vi "VL6180 Example.vi"() -> ()   [LabVIEW 2014]
uses:
  <vilib>/myRIO/Instrument Drivers/Onboard IO/DIO/typedefs/DIO Reference.ctl
  <vilib>/myRIO/Common/Instrument Driver Framework/Utilities/typedefs/myRIO Generic Hardware Reference.ctl
  <vilib>/myRIO/Common/Instrument Driver Framework/Utilities/typedefs/Hardware Version Enum.ctl
  <vilib>/myRIO/Common/Instrument Driver Framework/Utilities/typedefs/myRIO v1.0 Reference.ctl
  <vilib>/myRIO/Common/Instrument Driver Framework/Utilities/typedefs/Generic FPGA Reference.ctl
  <vilib>/myRIO/Common/Instrument Driver Framework/myRIO v1.0/DIO/typedefs/DIO Channels List.ctl
  <vilib>/myRIO/Common/Instrument Driver Framework/myRIO v1.0/DIO/typedefs/DIO Channels Enum.ctl
  <vilib>/userdefined/High Color/nirio_resource_hc.ctl
  <vilib>/myRIO/Common/Instrument Driver Framework/Utilities/vis/Is FPGA Ref Available.vi
  <vilib>/myRIO/Common/Instrument Driver Framework/myRIO v1.0/DIO/vis/myRIO v1.1 Open DIO.vi
  <vilib>/myRIO/Instrument Drivers/Onboard IO/DIO/vis/Write.vi
  <vilib>/myRIO/Common/Instrument Driver Framework/Utilities/vis/Validate Channels.vi
  <vilib>/myRIO/Common/Instrument Driver Framework/myRIO v1.0/DIO/vis/myRIO v1.0 Reserve DIO.vi
  <vilib>/myRIO/Common/Instrument Driver Framework/myRIO v1.0/Resource Manager/vis/myRIO v1.0 Reserve Channel List.vi
  <vilib>/myRIO/Common/Instrument Driver Framework/myRIO v1.0/DIO/vis/myRIO v1.0 Build MUX Configuration DIO.vi
  <vilib>/myRIO/Common/Instrument Driver Framework/myRIO v1.0/Resource Manager/vis/myRIO v1.0 Reserve Channel.vi
  <vilib>/myRIO/Common/Instrument Driver Framework/myRIO v1.0/Resource Manager/vis/myRIO v1.0 Unreserve Channel.vi
  <vilib>/myRIO/Common/Instrument Driver Framework/myRIO v1.0/Resource Manager/vis/myRIO v1.0 Create Configuration List.vi
  <vilib>/myRIO/Common/Instrument Driver Framework/myRIO v1.0/Resource Manager/vis/myRIO v1.0 Build Mutex Name.vi
  <vilib>/Utility/VariantDataType/GetNumericInfo.vi
  <vilib>/Utility/error.llb/Error Cluster From Error Code.vi
  <vilib>/myRIO/Common/Instrument Driver Framework/myRIO v1.0/myRIO v1.1 Open.vi
  <vilib>/myRIO/Common/Instrument Driver Framework/Utilities/vis/IO Manager.vi
  <vilib>/myRIO/Common/Instrument Driver Framework/Utilities/vis/Configuration Manager.vi
  <vilib>/myRIO/Common/Instrument Driver Framework/myRIO v1.0/Resource Manager/vis/myRIO v1.0 Configure IO.vi
  <vilib>/myRIO/Common/Instrument Driver Framework/myRIO v1.0/myRIO v1.0 Close.vi
  <vilib>/myRIO/Common/Instrument Driver Framework/myRIO v1.0/DIO/vis/myRIO v1.0 Write DIO.vi
  <vilib>/MakerHub/LINX/Public/Utilities/Open Local.vi
  <vilib>/myRIO/Express VI/Onboard IO/DO/DO Express VI.xnode
  <vilib>/myRIO/Instrument Drivers/Onboard IO/DIO/vis/myRIO DIO Open.xnode
  <vilib>/myRIO/Instrument Drivers/Onboard IO/DIO/DIO.lvlib
  <vilib>/MakerHub/LINX/LMH-LINX.lvlib
panel:
  in  "milliseconds to wait":u32
  in  "ToF 1 PWR":bool
  out "error out":errorcluster {"code" format="%.0x"}
  out "Sensor Error Code":u8
  out "Distance (mm)":u8
  in  "stop":bool
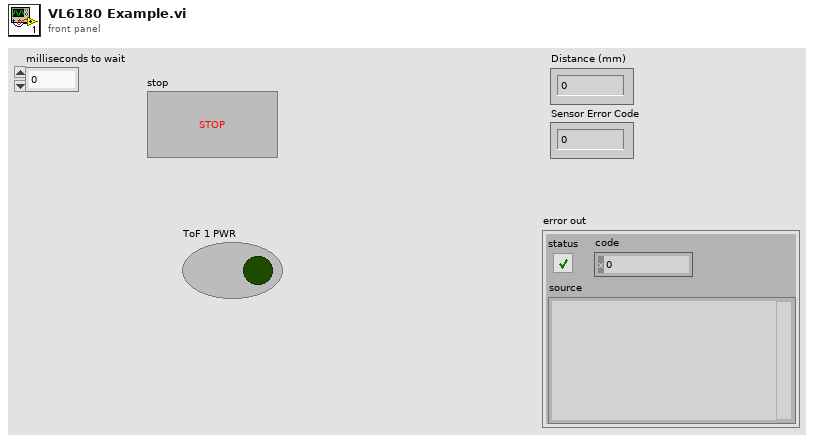
[diagram p1: front panel]
types:
  T1 = typedef "LMH-LINX.lvlib/LINX Ref.ctl" = cluster{"IO":T2, "Interface":T3, "LINX Device Config":T4}
  T2 = typedef "LMH-LINX.lvlib/Platform.ctl" = enum16{"Remote", "Local"}
  T3 = typedef "LMH-LINX.lvlib/Interface.ctl" = enum16{"Serial", "TCP"}
  T4 = typedef "LMH-LINX.lvlib/Device.lvlib/LINX Device Config.ctl" = cluster{"Interface":T3, "COM Port":refnum<visa-resource-name>, "TCP Configuration":T5, "Device Family":u8, "Device ID":u8, "Device Name":string, "TCP Ref":refnum<k5>, "Channels":T6}
  T5 = typedef "LMH-LINX.lvlib/Device.lvlib/TCP Config.ctl" = cluster{"IP Address":string, "Port":u16}
  T6 = typedef "LMH-LINX.lvlib/Channels.ctl" = cluster{"DI":u8[], "DO":u8[], "AI":u8[], "AO":u8[], "PWM":u8[], "QE":u8[], "UART":u8[], "I2C 2":u8[], "SPI":u8[], "CAN":u8[], "Servo":u8[], "AI Ref (V)":dbl, "AI Resolution (Bits)":u8, "AO Ref (V)":dbl, "AO Resolution (Bits)":u8}
  T7 = typedef "VL6180 Resource.ctl" = cluster{"I2C Channel":u8, "I2C Slave Address":u8, "Online":bool}
  T8 = typedef "DIO.lvlib/DIO Reference.ctl" = cluster{"myRIO Reference":T9, "DIO Channels List":T13}
  T9 = typedef "myRIO Generic Hardware Reference.ctl" = cluster{"myRIO Model":T10, "myRIO Hardware Reference":T11}
  T10 = typedef "Hardware Version Enum.ctl" = enum16{"Unknown", "myRIO-1900", "myRIO-1950"}
  T11 = typedef "myRIO v1.0 Reference.ctl" = cluster{"Generic FPGA Reference":T12, "Allow multiple opens":bool}
  T12 = typedef "Generic FPGA Reference.ctl" = refnum<k20>
  T13 = typedef "DIO Channels List.ctl" = T14[]
  T14 = typedef "DIO Channels Enum.ctl" = enum16{"Not Connected", "C/DIO0", "C/DIO1", "C/DIO2", "C/DIO3", "C/DIO4", "C/DIO5", "C/DIO6", "C/DIO7", "A/DIO0", "A/DIO1", "A/DIO2", "A/DIO3", "A/DIO4", "A/DIO5", "A/DIO6", "A/DIO7", "A/DIO8", "A/DIO9", "A/DIO10", "A/DIO11", "A/DIO12", "A/DIO13", "A/DIO14", "A/DIO15", "B/DIO0", "B/DIO1", "B/DIO2", "B/DIO3", "B/DIO4", "B/DIO5", "B/DIO6", "B/DIO7", "B/DIO8", "B/DIO9", "B/DIO10", "B/DIO11", "B/DIO12", "B/DIO13", "B/DIO14", "B/DIO15", "LED0", "LED1", "LED2", "LED3", "Button0"}
  T15 = typedef "nirio_resource_hc.ctl" = tag
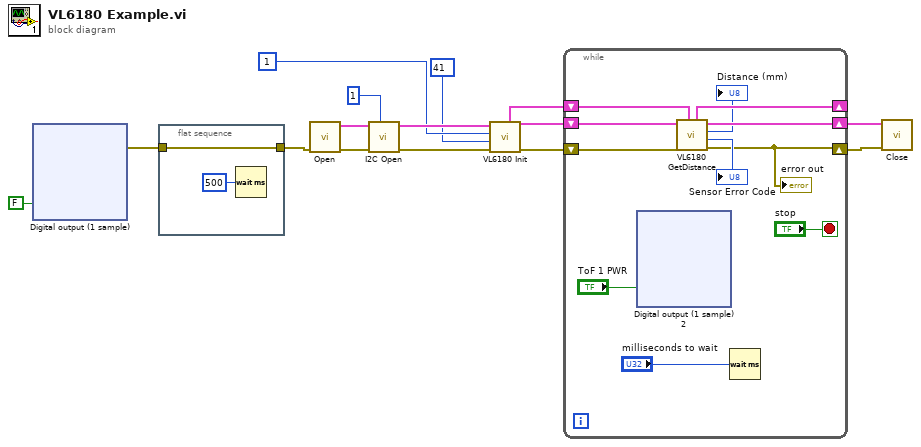
[diagram p0: block diagram]
diagram:
  n1 = xnode "Digital output (1 sample)"("ToF 1 PWR (B/DIO0 (Pin 11))"=FALSE ("ToF 1 PWR (A/DIO0 (Pin 11))")) -> ("error out"=w3:errorcluster)  [unwired: 1 in]
  n2 = flat-sequence {
    tunnel: [w17] -> w4
    tunnel: w3 -> [w17]
    frame #0 {
      n3 = Wait (ms)(milliseconds to wait=u32 500) -> ()  [unwired: 1 out]
    }
  }
  n4 = call-poly <vilib>:"Open.vi"("Error In"=w4) -> ("Error Out"=w15:errorcluster, "LINX Resource"=w14:T1)  [unwired: 8 in, 1 out]
  n5 = call <vilib>:"I2C Open.vi"("I2C Channel (0)"=u8 1, "Error In"=w15, "LINX Resource"=w14) -> ("Error Out"=w12:errorcluster, "LINX Resource"=w13:T1)  [unwired: 7 in]
  n6 = call "VL6180 Init.vi"("Error In"=w12, "I2C Slave Address"=u8 41, "I2C Channel"=u8 1 ("I2C Channel (0)"), "LINX Resource"=w13) -> ("Error Out"=w7:errorcluster, "LINX Resource"=w9:T1, "VL6180 Resource"=w8:T7)  [unwired: 5 in]
  n7 = while {
    shift-right: [w24] -> _
    shift-left: w8 -> [w26]
    shift-right: [w23] -> w6
    shift-left: w9 -> [w27]
    shift-right: [w20] -> w5
    shift-left: w7 -> [w25]
    stop <- "stop" stop-if-true
    n8 = xnode "Digital output (1 sample) 2"("ToF 1 PWR (B/DIO0 (Pin 11))"="ToF 1 PWR") -> ()  [unwired: 1 in, 1 out]
    n9 = call "VL6180 GetDistance.vi"("VL6180 Resource in"=w26, "error in (no error)"=w25, "LINX Resource"=w27) -> ("error out"=w20:errorcluster, "Sensor Error Code"=→"Sensor Error Code":u8, "Distance (mm)"=→"Distance (mm)":u8, "LINX Resource"=w23:T1, "VL6180 Resource out"=w24:T7)  [unwired: 3 in, 1 out]
    "error out" <- w20
    n10 = Wait (ms)(milliseconds to wait="milliseconds to wait") -> ()  [unwired: 1 out]
  }
  n11 = call <vilib>:"Close.vi"("Error In"=w5, "LINX Resource"=w6) -> ()  [unwired: 9 in, 1 out]
